vi "Dialog_TestBode (SubVI).vi"() -> ()   [LabVIEW 2017]
uses:
  <vilib>/Utility/miscctls.llb/LVRowAndColumnTypeDef.ctl
  Global_SNK3_HF.vi
panel:
  in  "Stop":bool
  in  "Clear":bool
  in  "FreqIndex":u32=46
  in  "FreqSel":bool
  in  "index":i32=11
  in  "Export":bool
  in  "Tab Control":enum32{"Page 1", "Page 2", "Page 3"}(tab)=enum."Page 2"
  in  "Table":string[][](table)=[["1.000000E+5", "1.000636E+5", "2.491840E-2"], ["1.120000E+5", "1.118741E+5", "3.785940E-2"], ["1.250000E+5", "1.249164E+5", "5.126945E-2"], ["1.400000E+5", "1.399830E+5", "6.506335E-2"], ["1.600000E+5", "1.599893E+5", "8.105153E-2"], ["1.800000E+5", "1.799900E+5", "9.492544E-2"], ["2.000000E+5", "1.999957E+5", "1.070040E-1"], ["2.240000E+5", "2.239947E+5", "1.194879E-1"], ["2.500000E+5", "2.499939E+5", "1.308049E-1"], ["2.800000E+5", "2.799909E+5", "1.415511E-1"], ["3.150000E+5", "3.149906E+5", "1.515264E-1"], ["3.550000E+5", "3.549888E+5", "1.604395E-1"], ["4.000000E+5", "3.999864E+5", "1.681297E-1"], ["4.500000E+5", "4.499863E+5", "1.745038E-1"], ["5.000000E+5", "4.999842E+5", "1.792983E-1"], ["5.600000E+5", "5.599829E+5", "1.838799E-1"], ["6.300000E+5", "6.299795E+5", "1.879248E-1"], ["7.100000E+5", "7.099802E+5", "1.908162E-1"], ["8.000000E+5", "7.999770E+5", "1.931713E-1"], ["9.000000E+5", "8.999726E+5", "1.950158E-1"], ["1.000000E+6", "9.999710E+5", "1.965268E-1"], ["1.120000E+6", "1.119965E+6", "1.976914E-1"], ["1.250000E+6", "1.249962E+6", "1.985237E-1"], ["1.400000E+6", "1.399956E+6", "1.991446E-1"], ["1.600000E+6", "1.599951E+6", "1.995656E-1"], ["1.800000E+6", "1.799943E+6", "1.997028E-1"], ["2.000000E+6", "1.999939E+6", "1.996953E-1"], ["2.240000E+6", "2.239928E+6", "1.994641E-1"], ["2.500000E+6", "2.499924E+6", "1.990983E-1"], ["2.800000E+6", "2.799912E+6", "1.985802E-1"], ["3.150000E+6", "3.149905E+6", "1.977598E-1"], ["3.550000E+6", "3.549890E+6", "1.967576E-1"], ["4.000000E+6", "3.999877E+6", "1.955042E-1"], ["4.500000E+6", "4.499864E+6", "1.940497E-1"], ["5.000000E+6", "4.999848E+6", "1.926097E-1"], ["5.600000E+6", "5.599830E+6", "1.907100E-1"], ["6.300000E+6", "6.299804E+6", "1.884695E-1"], ["7.100000E+6", "7.099783E+6", "1.857047E-1"], ["8.000000E+6", "7.999756E+6", "1.820427E-1"], ["9.000000E+6", "8.999724E+6", "1.769700E-1"], ["1.000000E+7", "9.999696E+6", "1.698254E-1"], ["1.120000E+7", "1.119966E+7", "1.575704E-1"], ["1.250000E+7", "1.249962E+7", "1.374566E-1"], ["1.400000E+7", "1.399957E+7", "1.010104E-1"], ["1.600000E+7", "1.599951E+7", "3.921273E-2"], ["1.800000E+7", "1.799945E+7", "7.166046E-3"], ["2.000000E+7", "1.999939E+7", "6.631099E-4"], ["1.000000E+5", "1.001610E+5", "2.507403E-2"], ["1.120000E+5", "1.118719E+5", "3.811099E-2"], ["1.250000E+5", "1.249126E+5", "5.159270E-2"], ["1.400000E+5", "1.399818E+5", "6.548660E-2"], ["1.600000E+5", "1.599863E+5", "8.150836E-2"], ["1.800000E+5", "1.799875E+5", "9.546910E-2"], ["2.000000E+5", "1.999953E+5", "1.076681E-1"], ["2.240000E+5", "2.239928E+5", "1.201877E-1"], ["2.500000E+5", "2.499918E+5", "1.316163E-1"], ["2.800000E+5", "2.799915E+5", "1.423784E-1"], ["3.150000E+5", "3.149935E+5", "1.525069E-1"], ["3.550000E+5", "3.549893E+5", "1.614557E-1"], ["4.000000E+5", "3.999897E+5", "1.690699E-1"], ["4.500000E+5", "4.499870E+5", "1.755943E-1"], ["5.000000E+5", "4.999845E+5", "1.803583E-1"], ["5.600000E+5", "5.599837E+5", "1.850528E-1"], ["6.300000E+5", "6.299822E+5", "1.891165E-1"], ["7.100000E+5", "7.099780E+5", "1.920091E-1"], ["8.000000E+5", "7.999766E+5", "1.943341E-1"], ["9.000000E+5", "8.999725E+5", "1.962455E-1"], ["1.000000E+6", "9.999694E+5", "1.977815E-1"], ["1.120000E+6", "1.119967E+6", "1.989120E-1"], ["1.250000E+6", "1.249961E+6", "1.997381E-1"], ["1.400000E+6", "1.399956E+6", "2.003866E-1"], ["1.600000E+6", "1.599951E+6", "2.008868E-1"], ["1.800000E+6", "1.799946E+6", "2.009867E-1"], ["2.000000E+6", "1.999937E+6", "2.010105E-1"], ["2.240000E+6", "2.239930E+6", "2.007797E-1"], ["2.500000E+6", "2.499926E+6", "2.004007E-1"], ["2.800000E+6", "2.799914E+6", "1.998448E-1"], ["3.150000E+6", "3.149906E+6", "1.990098E-1"], ["3.550000E+6", "3.549893E+6", "1.979898E-1"], ["4.000000E+6", "3.999878E+6", "1.966912E-1"], ["4.500000E+6", "4.499860E+6", "1.952348E-1"], ["5.000000E+6", "4.999849E+6", "1.936508E-1"], ["5.600000E+6", "5.599830E+6", "1.916568E-1"], ["6.300000E+6", "6.299805E+6", "1.893688E-1"], ["7.100000E+6", "7.099787E+6", "1.867505E-1"], ["8.000000E+6", "7.999758E+6", "1.838976E-1"], ["9.000000E+6", "8.999722E+6", "1.808635E-1"], ["1.000000E+7", "9.999696E+6", "1.777367E-1"], ["1.120000E+7", "1.119966E+7", "1.731531E-1"], ["1.250000E+7", "1.249962E+7", "1.649845E-1"], ["1.400000E+7", "1.399958E+7", "1.420928E-1"], ["1.600000E+7", "1.599951E+7", "7.711530E-2"], ["1.800000E+7", "1.799945E+7", "2.355849E-2"], ["2.000000E+7", "1.999939E+7", "4.626126E-3"], ["1.000000E+5", "1.001252E+5", "3.046975E-2"], ["1.120000E+5", "1.118759E+5", "4.637352E-2"], ["1.250000E+5", "1.249173E+5", "6.281049E-2"], ["1.400000E+5", "1.399846E+5", "7.988195E-2"], ["1.600000E+5", "1.599828E+5", "9.961572E-2"], ["1.800000E+5", "1.799853E+5", "1.168189E-1"], ["2.000000E+5", "1.999934E+5", "1.318127E-1"], ["2.240000E+5", "2.239952E+5", "1.473312E-1"], ["2.500000E+5", "2.499948E+5", "1.614577E-1"], ["2.800000E+5", "2.799918E+5", "1.749158E-1"], ["3.150000E+5", "3.149891E+5", "1.872912E-1"], ["3.550000E+5", "3.549888E+5", "1.983931E-1"], ["4.000000E+5", "3.999890E+5", "2.079678E-1"], ["4.500000E+5", "4.499874E+5", "2.159216E-1"], ["5.000000E+5", "4.999822E+5", "2.219795E-1"], ["5.600000E+5", "5.599815E+5", "2.277855E-1"], ["6.300000E+5", "6.299820E+5", "2.327026E-1"], ["7.100000E+5", "7.099788E+5", "2.362682E-1"], ["8.000000E+5", "7.999713E+5", "2.393311E-1"], ["9.000000E+5", "8.999711E+5", "2.416585E-1"], ["1.000000E+6", "9.999711E+5", "2.435690E-1"], ["1.120000E+6", "1.119965E+6", "2.450257E-1"], ["1.250000E+6", "1.249962E+6", "2.460204E-1"], ["1.400000E+6", "1.399956E+6", "2.467872E-1"], ["1.600000E+6", "1.599948E+6", "2.473571E-1"], ["1.800000E+6", "1.799945E+6", "2.475632E-1"], ["2.000000E+6", "1.999939E+6", "2.474866E-1"], ["2.240000E+6", "2.239933E+6", "2.470316E-1"], ["2.500000E+6", "2.499923E+6", "2.464084E-1"], ["2.800000E+6", "2.799913E+6", "2.454233E-1"], ["3.150000E+6", "3.149902E+6", "2.440672E-1"], ["3.550000E+6", "3.549894E+6", "2.421851E-1"], ["4.000000E+6", "3.999877E+6", "2.397798E-1"], ["4.500000E+6", "4.499864E+6", "2.368307E-1"], ["5.000000E+6", "4.999845E+6", "2.335615E-1"], ["5.600000E+6", "5.599827E+6", "2.292005E-1"], ["6.300000E+6", "6.299803E+6", "2.236615E-1"], ["7.100000E+6", "7.099783E+6", "2.165497E-1"], ["8.000000E+6", "7.999753E+6", "2.080278E-1"], ["9.000000E+6", "8.999724E+6", "1.978426E-1"], ["1.000000E+7", "9.999693E+6", "1.868804E-1"], ["1.120000E+7", "1.119965E+7", "1.725228E-1"], ["1.250000E+7", "1.249962E+7", "1.542881E-1"], ["1.400000E+7", "1.399957E+7", "1.237350E-1"], ["1.600000E+7", "1.599951E+7", "6.203397E-2"], ["1.800000E+7", "1.799944E+7", "1.812404E-2"], ["2.000000E+7", "1.999939E+7", "3.543936E-3"], ["1.000000E+5", "1.001588E+5", "2.947361E-2"], ["1.120000E+5", "1.118676E+5", "4.485788E-2"], ["1.250000E+5", "1.249118E+5", "6.086847E-2"], ["1.400000E+5", "1.399847E+5", "7.738364E-2"], ["1.600000E+5", "1.599909E+5", "9.659424E-2"], ["1.800000E+5", "1.799850E+5", "1.134125E-1"], ["2.000000E+5", "1.999928E+5", "1.281373E-1"], ["2.240000E+5", "2.239927E+5", "1.433162E-1"], ["2.500000E+5", "2.499955E+5", "1.571975E-1"], ["2.800000E+5", "2.799914E+5", "1.703684E-1"], ["3.150000E+5", "3.149886E+5", "1.827951E-1"], ["3.550000E+5", "3.549900E+5", "1.938016E-1"], ["4.000000E+5", "3.999887E+5", "2.034033E-1"], ["4.500000E+5", "4.499859E+5", "2.114272E-1"], ["5.000000E+5", "4.999831E+5", "2.175966E-1"], ["5.600000E+5", "5.599825E+5", "2.235053E-1"], ["6.300000E+5", "6.299793E+5", "2.287001E-1"], ["7.100000E+5", "7.099770E+5", "2.329029E-1"], ["8.000000E+5", "7.999752E+5", "2.365108E-1"], ["9.000000E+5", "8.999728E+5", "2.396521E-1"], ["1.000000E+6", "9.999702E+5", "2.422890E-1"], ["1.120000E+6", "1.119966E+6", "2.449885E-1"], ["1.250000E+6", "1.249961E+6", "2.474209E-1"], ["1.400000E+6", "1.399960E+6", "2.499920E-1"], ["1.600000E+6", "1.599951E+6", "2.531813E-1"], ["1.800000E+6", "1.799944E+6", "2.563808E-1"], ["2.000000E+6", "1.999939E+6", "2.597062E-1"], ["2.240000E+6", "2.239927E+6", "2.639021E-1"], ["2.500000E+6", "2.499924E+6", "2.688323E-1"], ["2.800000E+6", "2.799913E+6", "2.751680E-1"], ["3.150000E+6", "3.149904E+6", "2.834179E-1"], ["3.550000E+6", "3.549892E+6", "2.939424E-1"], ["4.000000E+6", "3.999879E+6", "3.073316E-1"], ["4.500000E+6", "4.499860E+6", "3.242399E-1"], ["5.000000E+6", "4.999846E+6", "3.430244E-1"], ["5.600000E+6", "5.599827E+6", "3.675444E-1"], ["6.300000E+6", "6.299807E+6", "3.977254E-1"], ["7.100000E+6", "7.099782E+6", "4.305227E-1"], ["8.000000E+6", "7.999753E+6", "4.582917E-1"], ["9.000000E+6", "8.999723E+6", "4.664814E-1"], ["1.000000E+7", "9.999692E+6", "4.421232E-1"], ["1.120000E+7", "1.119966E+7", "3.737524E-1"], ["1.250000E+7", "1.249961E+7", "2.750965E-1"], ["1.400000E+7", "1.399957E+7", "1.599110E-1"], ["1.600000E+7", "1.599950E+7", "4.612828E-2"], ["1.800000E+7", "1.799944E+7", "6.724351E-3"], ["2.000000E+7", "1.745191E+7", "5.547105E-4"], ["1.000000E+5", "1.001671E+5", "3.013311E-2"], ["1.120000E+5", "1.118716E+5", "4.587390E-2"], ["1.250000E+5", "1.249115E+5", "6.221882E-2"], ["1.400000E+5", "1.399901E+5", "7.910503E-2"], ["1.600000E+5", "1.599861E+5", "9.867014E-2"], ["1.800000E+5", "1.799875E+5", "1.157310E-1"], ["2.000000E+5", "1.999941E+5", "1.307408E-1"], ["2.240000E+5", "2.239941E+5", "1.461274E-1"], ["2.500000E+5", "2.499957E+5", "1.601914E-1"], ["2.800000E+5", "2.799922E+5", "1.735531E-1"], ["3.150000E+5", "3.149912E+5", "1.860088E-1"], ["3.550000E+5", "3.549891E+5", "1.971355E-1"], ["4.000000E+5", "3.999871E+5", "2.067383E-1"], ["4.500000E+5", "4.499858E+5", "2.147592E-1"], ["5.000000E+5", "4.999843E+5", "2.208970E-1"], ["5.600000E+5", "5.599830E+5", "2.267879E-1"], ["6.300000E+5", "6.299812E+5", "2.318491E-1"], ["7.100000E+5", "7.099781E+5", "2.356804E-1"], ["8.000000E+5", "7.999771E+5", "2.390532E-1"], ["9.000000E+5", "8.999704E+5", "2.418962E-1"], ["1.000000E+6", "9.999683E+5", "2.442224E-1"], ["1.120000E+6", "1.119965E+6", "2.463632E-1"], ["1.250000E+6", "1.249961E+6", "2.482126E-1"], ["1.400000E+6", "1.399956E+6", "2.498954E-1"], ["1.600000E+6", "1.599948E+6", "2.519791E-1"], ["1.800000E+6", "1.799946E+6", "2.538926E-1"], ["2.000000E+6", "1.999937E+6", "2.557256E-1"], ["2.240000E+6", "2.239932E+6", "2.579385E-1"], ["2.500000E+6", "2.499924E+6", "2.603118E-1"], ["2.800000E+6", "2.799913E+6", "2.634098E-1"], ["3.150000E+6", "3.149901E+6", "2.672305E-1"], ["3.550000E+6", "3.549891E+6", "2.720161E-1"], ["4.000000E+6", "3.999873E+6", "2.780268E-1"], ["4.500000E+6", "4.499860E+6", "2.852321E-1"], ["5.000000E+6", "4.999845E+6", "2.930384E-1"], ["5.600000E+6", "5.599826E+6", "3.028215E-1"], ["6.300000E+6", "6.299804E+6", "3.141354E-1"], ["7.100000E+6", "7.099781E+6", "3.257264E-1"], ["8.000000E+6", "7.999753E+6", "3.345783E-1"], ["9.000000E+6", "8.999721E+6", "3.357425E-1"], ["1.000000E+7", "9.999692E+6", "3.236355E-1"], ["1.120000E+7", "1.119965E+7", "2.898888E-1"], ["1.250000E+7", "1.249961E+7", "2.321748E-1"], ["1.400000E+7", "1.399957E+7", "1.483795E-1"], ["1.600000E+7", "1.599951E+7", "4.683820E-2"], ["1.800000E+7", "1.799944E+7", "7.169091E-3"], ["2.000000E+7", "1.999938E+7", "5.872768E-4"], ["1.000000E+5", "1.001573E+5", "3.042811E-2"], ["1.120000E+5", "1.118676E+5", "4.631044E-2"], ["1.250000E+5", "1.249112E+5", "6.278921E-2"], ["1.400000E+5", "1.399824E+5", "7.977333E-2"], ["1.600000E+5", "1.599897E+5", "9.949145E-2"], ["1.800000E+5", "1.799905E+5", "1.167352E-1"], ["2.000000E+5", "1.999960E+5", "1.317144E-1"], ["2.240000E+5", "2.239941E+5", "1.472570E-1"], ["2.500000E+5", "2.499914E+5", "1.614052E-1"], ["2.800000E+5", "2.799928E+5", "1.747607E-1"], ["3.150000E+5", "3.149895E+5", "1.872958E-1"], ["3.550000E+5", "3.549889E+5", "1.984372E-1"], ["4.000000E+5", "3.999899E+5", "2.080880E-1"], ["4.500000E+5", "4.499863E+5", "2.160420E-1"], ["5.000000E+5", "4.999824E+5", "2.221527E-1"], ["5.600000E+5", "5.599829E+5", "2.279609E-1"], ["6.300000E+5", "6.299811E+5", "2.329477E-1"], ["7.100000E+5", "7.099769E+5", "2.367245E-1"], ["8.000000E+5", "7.999745E+5", "2.398766E-1"], ["9.000000E+5", "8.999738E+5", "2.424630E-1"], ["1.000000E+6", "9.999694E+5", "2.445476E-1"], ["1.120000E+6", "1.119967E+6", "2.463587E-1"], ["1.250000E+6", "1.249961E+6", "2.477818E-1"], ["1.400000E+6", "1.399959E+6", "2.489776E-1"], ["1.600000E+6", "1.599947E+6", "2.503258E-1"], ["1.800000E+6", "1.799945E+6", "2.512193E-1"], ["2.000000E+6", "1.999942E+6", "2.520426E-1"], ["2.240000E+6", "2.239932E+6", "2.529437E-1"], ["2.500000E+6", "2.499923E+6", "2.538312E-1"], ["2.800000E+6", "2.799913E+6", "2.548656E-1"], ["3.150000E+6", "3.149903E+6", "2.559440E-1"], ["3.550000E+6", "3.549890E+6", "2.573163E-1"], ["4.000000E+6", "3.999877E+6", "2.589801E-1"], ["4.500000E+6", "4.499858E+6", "2.609782E-1"], ["5.000000E+6", "4.999846E+6", "2.630935E-1"], ["5.600000E+6", "5.599829E+6", "2.654121E-1"], ["6.300000E+6", "6.299805E+6", "2.678989E-1"], ["7.100000E+6", "7.099784E+6", "2.696164E-1"], ["8.000000E+6", "7.999755E+6", "2.688480E-1"], ["9.000000E+6", "8.999722E+6", "2.633041E-1"], ["1.000000E+7", "9.999690E+6", "2.505779E-1"], ["1.120000E+7", "1.119966E+7", "2.241202E-1"], ["1.250000E+7", "1.249961E+7", "1.824472E-1"], ["1.400000E+7", "1.399957E+7", "1.204614E-1"], ["1.600000E+7", "1.599951E+7", "4.016119E-2"], ["1.800000E+7", "1.799944E+7", "6.498026E-3"], ["2.000000E+7", "1.999938E+7", "5.582479E-4"], ["1.000000E+5", "1.001346E+5", "3.073302E-2"], ["1.120000E+5", "1.118727E+5", "4.677344E-2"], ["1.250000E+5", "1.249160E+5", "6.336208E-2"], ["1.400000E+5", "1.399837E+5", "8.046874E-2"], ["1.600000E+5", "1.599845E+5", "1.003864E-1"], ["1.800000E+5", "1.799893E+5", "1.177135E-1"], ["2.000000E+5", "1.999962E+5", "1.328408E-1"], ["2.240000E+5", "2.239946E+5", "1.484407E-1"], ["2.500000E+5", "2.499937E+5", "1.626519E-1"], ["2.800000E+5", "2.799899E+5", "1.761700E-1"], ["3.150000E+5", "3.149904E+5", "1.887583E-1"], ["3.550000E+5", "3.549888E+5", "1.998843E-1"], ["4.000000E+5", "3.999893E+5", "2.095560E-1"], ["4.500000E+5", "4.499866E+5", "2.176090E-1"], ["5.000000E+5", "4.999851E+5", "2.236199E-1"], ["5.600000E+5", "5.599840E+5", "2.295974E-1"], ["6.300000E+5", "6.299794E+5", "2.345735E-1"], ["7.100000E+5", "7.099800E+5", "2.382895E-1"], ["8.000000E+5", "7.999734E+5", "2.415122E-1"], ["9.000000E+5", "8.999709E+5", "2.440727E-1"], ["1.000000E+6", "9.999682E+5", "2.462285E-1"], ["1.120000E+6", "1.119965E+6", "2.480292E-1"], ["1.250000E+6", "1.249961E+6", "2.494651E-1"], ["1.400000E+6", "1.399958E+6", "2.506996E-1"], ["1.600000E+6", "1.599950E+6", "2.518965E-1"], ["1.800000E+6", "1.799947E+6", "2.529126E-1"], ["2.000000E+6", "1.999942E+6", "2.536920E-1"], ["2.240000E+6", "2.239931E+6", "2.547042E-1"], ["2.500000E+6", "2.499926E+6", "2.555771E-1"], ["2.800000E+6", "2.799914E+6", "2.565540E-1"], ["3.150000E+6", "3.149903E+6", "2.577524E-1"], ["3.550000E+6", "3.549891E+6", "2.590071E-1"], ["4.000000E+6", "3.999877E+6", "2.606799E-1"], ["4.500000E+6", "4.499863E+6", "2.625431E-1"], ["5.000000E+6", "4.999848E+6", "2.645213E-1"], ["5.600000E+6", "5.599827E+6", "2.667418E-1"], ["6.300000E+6", "6.299808E+6", "2.690356E-1"], ["7.100000E+6", "7.099784E+6", "2.709912E-1"], ["8.000000E+6", "7.999756E+6", "2.714708E-1"], ["9.000000E+6", "8.999725E+6", "2.690780E-1"], ["1.000000E+7", "9.999694E+6", "2.619751E-1"], ["1.120000E+7", "1.119966E+7", "2.461795E-1"], ["1.250000E+7", "1.249962E+7", "2.187268E-1"], ["1.400000E+7", "1.399957E+7", "1.694056E-1"], ["1.600000E+7", "1.599951E+7", "7.900056E-2"], ["1.800000E+7", "1.799946E+7", "2.134967E-2"], ["2.000000E+7", "1.999939E+7", "3.896080E-3"], ["1.000000E+5", "7.271622E+6", "3.725159E-4"], ["1.120000E+5", "8.112799E+6", "3.764415E-4"], ["1.250000E+5", "7.224727E+6", "3.662772E-4"], ["1.400000E+5", "7.308552E+6", "3.973020E-4"], ["1.600000E+5", "4.309535E+6", "3.626683E-4"], ["1.800000E+5", "6.453873E+6", "3.560410E-4"], ["2.000000E+5", "5.085443E+6", "3.513905E-4"], ["2.240000E+5", "7.989710E+6", "3.810558E-4"], ["2.500000E+5", "6.352418E+6", "3.677376E-4"], ["2.800000E+5", "7.506742E+6", "3.607153E-4"], ["3.150000E+5", "6.668509E+6", "3.890383E-4"], ["3.550000E+5", "6.895082E+6", "3.819765E-4"], ["4.000000E+5", "6.273636E+6", "3.413821E-4"], ["4.500000E+5", "6.840624E+6", "3.723358E-4"], ["5.000000E+5", "5.049030E+6", "3.681375E-4"], ["5.600000E+5", "6.333587E+6", "3.807082E-4"], ["6.300000E+5", "7.345420E+6", "3.871347E-4"], ["7.100000E+5", "7.099786E+5", "2.374579E-1"], ["8.000000E+5", "7.999729E+5", "2.406560E-1"], ["9.000000E+5", "8.999716E+5", "2.431850E-1"], ["1.000000E+6", "9.999691E+5", "2.451838E-1"], ["1.120000E+6", "1.119965E+6", "2.469041E-1"], ["1.250000E+6", "1.249961E+6", "2.482266E-1"], ["1.400000E+6", "1.399956E+6", "2.493007E-1"], ["1.600000E+6", "1.599949E+6", "2.503615E-1"], ["1.800000E+6", "1.799944E+6", "2.510987E-1"], ["2.000000E+6", "1.999940E+6", "2.517382E-1"], ["2.240000E+6", "2.239928E+6", "2.522363E-1"], ["2.500000E+6", "2.499921E+6", "2.527697E-1"], ["2.800000E+6", "2.799912E+6", "2.533518E-1"], ["3.150000E+6", "3.149900E+6", "2.538616E-1"], ["3.550000E+6", "3.549889E+6", "2.545760E-1"], ["4.000000E+6", "3.999879E+6", "2.551996E-1"], ["4.500000E+6", "4.499862E+6", "2.559211E-1"], ["5.000000E+6", "4.999847E+6", "2.566902E-1"], ["5.600000E+6", "5.599826E+6", "2.574986E-1"], ["6.300000E+6", "6.299806E+6", "2.578567E-1"], ["7.100000E+6", "7.099781E+6", "2.571842E-1"], ["8.000000E+6", "7.999755E+6", "2.542991E-1"], ["9.000000E+6", "8.999722E+6", "2.471375E-1"], ["1.000000E+7", "9.999692E+6", "2.341935E-1"], ["1.120000E+7", "1.119965E+7", "2.099252E-1"], ["1.250000E+7", "1.249961E+7", "1.724919E-1"], ["1.400000E+7", "1.399957E+7", "1.158079E-1"], ["1.600000E+7", "1.599951E+7", "3.952577E-2"], ["1.800000E+7", "1.799944E+7", "6.504605E-3"], ["2.000000E+7", "1.999938E+7", "5.650367E-4"], ["1.000000E+5", "1.001674E+5", "3.072473E-2"], ["1.120000E+5", "1.118718E+5", "4.674261E-2"], ["1.250000E+5", "1.249089E+5", "6.334272E-2"], ["1.400000E+5", "1.399846E+5", "8.047815E-2"], ["1.600000E+5", "1.599821E+5", "1.003712E-1"], ["1.800000E+5", "1.799898E+5", "1.176893E-1"], ["2.000000E+5", "1.999934E+5", "1.327762E-1"], ["2.240000E+5", "2.239896E+5", "1.483583E-1"], ["2.500000E+5", "2.499930E+5", "1.626360E-1"], ["2.800000E+5", "2.799919E+5", "1.760684E-1"], ["3.150000E+5", "3.149892E+5", "1.886214E-1"], ["3.550000E+5", "3.549895E+5", "1.997476E-1"], ["4.000000E+5", "3.999900E+5", "2.094032E-1"], ["4.500000E+5", "4.499880E+5", "2.174488E-1"], ["5.000000E+5", "4.999829E+5", "2.235411E-1"], ["5.600000E+5", "5.599852E+5", "2.293669E-1"], ["6.300000E+5", "6.299816E+5", "2.344044E-1"], ["7.100000E+5", "7.099792E+5", "2.380854E-1"], ["8.000000E+5", "7.999787E+5", "2.411883E-1"], ["9.000000E+5", "8.999727E+5", "2.436654E-1"], ["1.000000E+6", "9.999702E+5", "2.457231E-1"], ["1.120000E+6", "1.119968E+6", "2.474353E-1"], ["1.250000E+6", "1.249962E+6", "2.487468E-1"], ["1.400000E+6", "1.399959E+6", "2.498615E-1"], ["1.600000E+6", "1.599952E+6", "2.508693E-1"], ["1.800000E+6", "1.799943E+6", "2.517389E-1"], ["2.000000E+6", "1.999941E+6", "2.522760E-1"], ["2.240000E+6", "2.239933E+6", "2.527969E-1"], ["2.500000E+6", "2.499923E+6", "2.533575E-1"], ["2.800000E+6", "2.799916E+6", "2.538892E-1"], ["3.150000E+6", "3.149903E+6", "2.544033E-1"], ["3.550000E+6", "3.549890E+6", "2.550274E-1"], ["4.000000E+6", "3.999878E+6", "2.557525E-1"], ["4.500000E+6", "4.499865E+6", "2.565297E-1"], ["5.000000E+6", "4.999845E+6", "2.572363E-1"], ["5.600000E+6", "5.599828E+6", "2.580387E-1"], ["6.300000E+6", "6.299804E+6", "2.584150E-1"], ["7.100000E+6", "7.099784E+6", "2.577035E-1"], ["8.000000E+6", "7.999757E+6", "2.547739E-1"], ["9.000000E+6", "8.999726E+6", "2.475172E-1"], ["1.000000E+7", "9.999692E+6", "2.346899E-1"], ["1.120000E+7", "1.119966E+7", "2.102803E-1"], ["1.250000E+7", "1.249962E+7", "1.727500E-1"], ["1.400000E+7", "1.399957E+7", "1.159860E-1"], ["1.600000E+7", "1.599951E+7", "3.956788E-2"], ["1.800000E+7", "1.799945E+7", "6.511833E-3"], ["2.000000E+7", "1.999939E+7", "5.656747E-4"], ["1.000000E+5", "4.945255E+6", "3.784724E-4"], ["1.120000E+5", "6.375661E+6", "3.745710E-4"], ["1.250000E+5", "1.250073E+5", "6.132748E-4"], ["1.400000E+5", "1.399781E+5", "1.172522E-3"], ["1.600000E+5", "1.600019E+5", "2.449967E-3"], ["1.800000E+5", "1.799905E+5", "4.581770E-3"], ["2.000000E+5", "1.999999E+5", "7.885116E-3"], ["2.240000E+5", "2.240013E+5", "1.387170E-2"], ["2.500000E+5", "2.499991E+5", "2.357577E-2"], ["2.800000E+5", "2.799918E+5", "3.982715E-2"], ["3.150000E+5", "3.149929E+5", "6.635508E-2"], ["3.550000E+5", "3.549946E+5", "1.045620E-1"], ["4.000000E+5", "3.999874E+5", "1.487510E-1"], ["4.500000E+5", "4.499825E+5", "1.863709E-1"], ["5.000000E+5", "4.999817E+5", "2.090956E-1"], ["5.600000E+5", "5.599827E+5", "2.239868E-1"], ["6.300000E+5", "6.299815E+5", "2.330744E-1"], ["7.100000E+5", "7.099780E+5", "2.383611E-1"], ["8.000000E+5", "7.999752E+5", "2.420167E-1"], ["9.000000E+5", "8.999734E+5", "2.447763E-1"], ["1.000000E+6", "9.999693E+5", "2.468706E-1"], ["1.120000E+6", "1.119966E+6", "2.485843E-1"], ["1.250000E+6", "1.249960E+6", "2.498993E-1"], ["1.400000E+6", "1.399960E+6", "2.509156E-1"], ["1.600000E+6", "1.599954E+6", "2.521203E-1"], ["1.800000E+6", "1.799947E+6", "2.528407E-1"], ["2.000000E+6", "1.999941E+6", "2.534274E-1"], ["2.240000E+6", "2.239932E+6", "2.540286E-1"], ["2.500000E+6", "2.499922E+6", "2.545439E-1"], ["2.800000E+6", "2.799913E+6", "2.550617E-1"], ["3.150000E+6", "3.149905E+6", "2.555762E-1"], ["3.550000E+6", "3.549890E+6", "2.562070E-1"], ["4.000000E+6", "3.999879E+6", "2.568503E-1"], ["4.500000E+6", "4.499863E+6", "2.576394E-1"], ["5.000000E+6", "4.999848E+6", "2.583673E-1"], ["5.600000E+6", "5.599828E+6", "2.590441E-1"], ["6.300000E+6", "6.299811E+6", "2.594208E-1"], ["7.100000E+6", "7.099782E+6", "2.587419E-1"], ["8.000000E+6", "7.999757E+6", "2.556978E-1"], ["9.000000E+6", "8.999729E+6", "2.484300E-1"], ["1.000000E+7", "9.999696E+6", "2.355078E-1"], ["1.120000E+7", "1.119966E+7", "2.112248E-1"], ["1.250000E+7", "1.249962E+7", "1.739360E-1"], ["1.400000E+7", "1.399957E+7", "1.167797E-1"], ["1.600000E+7", "1.599951E+7", "3.926693E-2"], ["1.800000E+7", "1.799945E+7", "6.325551E-3"], ["2.000000E+7", "1.999939E+7", "5.422671E-4"], ["1.000000E+5", "6.172924E+6", "3.758029E-4"], ["1.120000E+5", "5.205844E+6", "3.767627E-4"], ["1.250000E+5", "1.250007E+5", "6.162397E-4"], ["1.400000E+5", "1.399804E+5", "1.177858E-3"], ["1.600000E+5", "1.600003E+5", "2.461317E-3"], ["1.800000E+5", "1.799938E+5", "4.602202E-3"], ["2.000000E+5", "2.000005E+5", "7.917076E-3"], ["2.240000E+5", "2.239992E+5", "1.394228E-2"], ["2.500000E+5", "2.499997E+5", "2.367325E-2"], ["2.800000E+5", "2.799971E+5", "4.000153E-2"], ["3.150000E+5", "3.149938E+5", "6.665400E-2"], ["3.550000E+5", "3.549936E+5", "1.050529E-1"], ["4.000000E+5", "3.999878E+5", "1.493885E-1"], ["4.500000E+5", "4.499854E+5", "1.871373E-1"], ["5.000000E+5", "4.999850E+5", "2.099204E-1"], ["5.600000E+5", "5.599840E+5", "2.249705E-1"], ["6.300000E+5", "6.299796E+5", "2.340463E-1"], ["7.100000E+5", "7.099780E+5", "2.393587E-1"], ["8.000000E+5", "7.999747E+5", "2.431090E-1"], ["9.000000E+5", "8.999714E+5", "2.458491E-1"], ["1.000000E+6", "9.999705E+5", "2.479870E-1"], ["1.120000E+6", "1.119964E+6", "2.496587E-1"], ["1.250000E+6", "1.249962E+6", "2.510589E-1"], ["1.400000E+6", "1.399958E+6", "2.521599E-1"], ["1.600000E+6", "1.599952E+6", "2.532737E-1"], ["1.800000E+6", "1.799945E+6", "2.541091E-1"], ["2.000000E+6", "1.999939E+6", "2.546832E-1"], ["2.240000E+6", "2.239931E+6", "2.552231E-1"], ["2.500000E+6", "2.499922E+6", "2.557674E-1"], ["2.800000E+6", "2.799916E+6", "2.562845E-1"], ["3.150000E+6", "3.149902E+6", "2.569137E-1"], ["3.550000E+6", "3.549892E+6", "2.574992E-1"], ["4.000000E+6", "3.999881E+6", "2.581088E-1"], ["4.500000E+6", "4.499866E+6", "2.587312E-1"], ["5.000000E+6", "4.999849E+6", "2.594061E-1"], ["5.600000E+6", "5.599830E+6", "2.599108E-1"], ["6.300000E+6", "6.299809E+6", "2.602532E-1"], ["7.100000E+6", "7.099784E+6", "2.598564E-1"], ["8.000000E+6", "7.999759E+6", "2.578969E-1"], ["9.000000E+6", "8.999725E+6", "2.536606E-1"], ["1.000000E+7", "9.999695E+6", "2.460182E-1"], ["1.120000E+7", "1.119966E+7", "2.318706E-1"], ["1.250000E+7", "1.249962E+7", "2.082904E-1"], ["1.400000E+7", "1.399957E+7", "1.640904E-1"], ["1.600000E+7", "1.599951E+7", "7.713568E-2"], ["1.800000E+7", "1.799945E+7", "2.076200E-2"], ["2.000000E+7", "1.999939E+7", "3.781710E-3"]]
  out "XY Graph - Light":cluster{dbl[], dbl[]}[](graph)=[{[100000.0], [-32.06959712907717]}, {[111999.99999999999, 125000.0, 140000.0, 160000.0, 180000.0, 200000.0, 223999.99999999997, 250000.0, 280000.0, 315000.0, 355000.0, 400000.0, 450000.0, 500000.0, 560000.0, 630000.0, 710000.0, 800000.0, 900000.0, 1000000.0, 1119999.9999999998, 1250000.0, 1400000.0, 1600000.0, 1800000.0, 2000000.0, 2239999.9999999995, 2500000.0, 2800000.0, 3150000.0, 3550000.0, 4000000.0, 4500000.0, 5000000.0, 5600000.0, 6300000.0, 7100000.0, 8000000.0, 9000000.0, 10000000.0, 11199999.999999998, 12500000.0, 14000000.0, 16000000.0, 18000000.0, 20000000.0], [-28.436526298205948, -25.802826263296893, -23.7332719575054, -21.82477578258775, -20.452347258891514, -19.412002724486356, -18.45351884411941, -17.667519012682238, -16.98173568676242, -16.390231995354895, -15.893775113201198, -15.487111701662231, -15.16390087209189, -14.928475216865047, -14.709313208203444, -14.52032036334469, -14.387693344743568, -14.281150043223814, -14.198605408554283, -14.131565591838937, -14.08024587698728, -14.043750917215725, -14.016628526957223, -13.998285225401968, -13.992317823456125, -13.992641918238395, -14.002703149579682, -14.018650076231129, -14.04128269413424, -14.077239595490907, -14.121370204146462, -14.176878604262049, -14.241741662590712, -14.306437043319807, -14.392531267070934, -14.495179556946546, -14.623544203236058, -14.796536706787954, -15.042006383001034, -15.399947629850084, -16.050507306854122, -17.23668939060284, -19.912677810583506, -28.131459030407164, -42.89440763935011, -63.56829035942]}, {[100000.0, 111999.99999999999, 125000.0, 140000.0, 160000.0, 180000.0, 200000.0, 223999.99999999997, 250000.0, 280000.0, 315000.0, 355000.0, 400000.0, 450000.0, 500000.0, 560000.0, 630000.0, 710000.0, 800000.0, 900000.0, 1000000.0, 1119999.9999999998, 1250000.0, 1400000.0, 1600000.0, 1800000.0, 2000000.0, 2239999.9999999995, 2500000.0, 2800000.0, 3150000.0, 3550000.0, 4000000.0, 4500000.0, 5000000.0, 5600000.0, 6300000.0, 7100000.0, 8000000.0, 9000000.0, 10000000.0, 11199999.999999998, 12500000.0, 14000000.0, 16000000.0, 18000000.0, 20000000.0], [-32.01551889429962, -28.37899452707971, -25.74823483212413, -23.676951031879764, -21.77595640844784, -20.40274326154021, -19.358259454411325, -18.402801613986824, -17.613805446903246, -16.93111990056153, -16.33421225385209, -15.838929891678752, -15.438674054644316, -15.109793842110058, -14.877276187309834, -14.65408910002438, -14.46541001449438, -14.333564100378442, -14.2290213916183, -14.144008009132534, -14.076285861022662, -14.026778773392161, -13.990782390455067, -13.962626095388547, -13.940972167945166, -13.936653414445281, -13.93562605041957, -13.945605110001921, -13.962017482691687, -13.986141635395718, -14.022512471882182, -14.067143854670874, -14.124299218352473, -14.188853652759148, -14.259612495960825, -14.349517323308962, -14.453830406996547, -14.574765674860101, -14.708480691090395, -14.852983060476303, -15.004455418435583, -15.23139293918094, -15.651137537678274, -16.948557340120082, -22.257188494263005, -32.557051745684504, -46.69565079423197]}, {[100000.0, 111999.99999999999, 125000.0, 140000.0, 160000.0, 180000.0, 200000.0, 223999.99999999997, 250000.0, 280000.0, 315000.0, 355000.0, 400000.0, 450000.0, 500000.0, 560000.0, 630000.0, 710000.0, 800000.0, 900000.0, 1000000.0, 1119999.9999999998, 1250000.0, 1400000.0, 1600000.0, 1800000.0, 2000000.0, 2239999.9999999995, 2500000.0, 2800000.0, 3150000.0, 3550000.0, 4000000.0, 4500000.0, 5000000.0, 5600000.0, 6300000.0, 7100000.0, 8000000.0, 9000000.0, 10000000.0, 11199999.999999998, 12500000.0, 14000000.0, 16000000.0, 18000000.0, 20000000.0], [-30.322621218434477, -26.674599312380135, -24.039355742967786, -21.951026345450444, -20.033442386519425, -18.64973877846673, -17.600856535055836, -16.63410559857063, -15.83882726130537, -15.143417277389128, -14.549652554538168, -14.049467339340184, -13.6400770187213, -13.314077380890701, -13.073743856192044, -12.849477273241554, -12.663977095040204, -12.531894145111133, -12.420015799221297, -12.33595721749724, -12.267560469194702, -12.215768532393055, -12.180579015082117, -12.153546074218175, -12.133510861761497, -12.12627824947159, -12.128967694603269, -12.144950624208512, -12.166889105606614, -12.201685155510308, -12.249811738460137, -12.317053271217207, -12.403748427428795, -12.511239170989356, -12.631974094798718, -12.795689318081582, -13.008175123698402, -13.288846918372247, -13.637571959268593, -14.073604548608769, -14.56872406173578, -15.26306825122991, -16.233350560286397, -18.150148684410517, -24.147407966054967, -34.83489953792064, -49.010283136140494]}, {[100000.0, 111999.99999999999, 125000.0, 140000.0, 160000.0, 180000.0, 200000.0, 223999.99999999997, 250000.0, 280000.0, 315000.0, 355000.0, 400000.0, 450000.0, 500000.0, 560000.0, 630000.0, 710000.0, 800000.0, 900000.0, 1000000.0, 1119999.9999999998, 1250000.0, 1400000.0, 1600000.0, 1800000.0, 2000000.0, 2239999.9999999995, 2500000.0, 2800000.0, 3150000.0, 3550000.0, 4000000.0, 4500000.0, 5000000.0, 5600000.0, 6300000.0, 7100000.0, 8000000.0, 9000000.0, 10000000.0, 11199999.999999998, 12500000.0, 14000000.0, 16000000.0, 18000000.0, 20000000.0], [-30.61133369738789, -26.963226015672408, -24.312152300260493, -22.22701720360909, -20.30097563747857, -18.90678532691976, -17.846487376256462, -16.874093584233275, -16.071085496798904, -15.372220087819837, -14.760709193608438, -14.252851833614361, -13.832841107089678, -13.496784135647319, -13.246958490658088, -13.01424181279698, -12.81467178595403, -12.656501341972826, -12.522979917934427, -12.408375492365128, -12.313327623976056, -12.21708601380307, -12.131271682782272, -12.04147663588503, -11.931368786082132, -11.822288890386137, -11.710354665088174, -11.571143527779846, -11.410370324688335, -11.208041474378902, -10.951453674000465, -10.634756112896229, -10.247856230096259, -9.782671188369868, -9.293500006339334, -8.69380341275508, -8.008333928935542, -7.320078807085363, -6.777160551500607, -6.623312531960201, -7.089134809418943, -8.548319619608288, -11.21029715297354, -15.922431897186373, -26.720654327600442, -43.446992917597, -65.11867214507339]}, {[100000.0, 111999.99999999999, 125000.0, 140000.0, 160000.0, 180000.0, 200000.0, 223999.99999999997, 250000.0, 280000.0, 315000.0, 355000.0, 400000.0, 450000.0, 500000.0, 560000.0, 630000.0, 710000.0, 800000.0, 900000.0, 1000000.0, 1119999.9999999998, 1250000.0, 1400000.0, 1600000.0, 1800000.0, 2000000.0, 2239999.9999999995, 2500000.0, 2800000.0, 3150000.0, 3550000.0, 4000000.0, 4500000.0, 5000000.0, 5600000.0, 6300000.0, 7100000.0, 8000000.0, 9000000.0, 10000000.0, 11199999.999999998, 12500000.0, 14000000.0, 16000000.0, 18000000.0, 20000000.0], [-30.41912035321658, -26.768686854286035, -24.121564852930433, -22.035918034919998, -20.11628492359509, -18.731007508690304, -17.67178020513984, -16.705366019589768, -15.907216887832798, -15.21135159574845, -14.609327938842513, -14.10470130853527, -13.691582339358213, -13.360964284671827, -13.116205469885676, -12.887600720975048, -12.695892003681614, -12.553529436783348, -12.430110309952902, -12.32741743046304, -12.244288567857806, -12.168483384389607, -12.103522164856294, -12.044833880465378, -11.972709681316775, -11.907000406404599, -11.844515582541694, -11.769675619461665, -11.690123894865298, -11.587361772358634, -11.462278975379236, -11.308107441500576, -11.118265772506817, -10.896031225741762, -10.661508462404504, -10.376264686527499, -10.057661589904734, -9.742940895315584, -9.510045715933911, -9.479873007304905, -9.798877177842863, -10.755370700425487, -12.683696600970704, -16.57252108145334, -26.587996933968444, -42.8907183233943, -64.62314271153984]}, {[100000.0, 111999.99999999999, 125000.0, 140000.0, 160000.0, 180000.0, 200000.0, 223999.99999999997, 250000.0, 280000.0, 315000.0, 355000.0, 400000.0, 450000.0, 500000.0, 560000.0, 630000.0, 710000.0, 800000.0, 900000.0, 1000000.0, 1119999.9999999998, 1250000.0, 1400000.0, 1600000.0, 1800000.0, 2000000.0, 2239999.9999999995, 2500000.0, 2800000.0, 3150000.0, 3550000.0, 4000000.0, 4500000.0, 5000000.0, 5600000.0, 6300000.0, 7100000.0, 8000000.0, 9000000.0, 10000000.0, 11199999.999999998, 12500000.0, 14000000.0, 16000000.0, 18000000.0, 20000000.0], [-30.33450156596599, -26.686421458352868, -24.042299781442434, -21.96284517278093, -20.04428464259955, -18.655966429280745, -17.60733470043496, -16.638479338035044, -15.841648411980444, -15.15112442170788, -14.549438867976725, -14.047538572712, -13.635058488279245, -13.309234710302002, -13.066969241980635, -12.84279115991943, -12.654833198920299, -12.515134570073972, -12.400243590644633, -12.30709032840063, -12.232731212616173, -12.168643308975236, -12.118612808408507, -12.07679605908064, -12.02988614388056, -11.998938644551348, -11.970521047293492, -11.939523834626698, -11.909099785768307, -11.873774674735621, -11.83710084124488, -11.790653095959714, -11.734672393853796, -11.667914202761203, -11.597796461965483, -11.521584980850847, -11.440581004281576, -11.38507545220435, -11.409864067646199, -11.590848492118708, -12.021146340221676, -12.990378844603033, -14.777256627783688, -18.383044645435472, -27.923869003228216, -43.744371659949636, -65.06345806592672]}, {[100000.0, 111999.99999999999, 125000.0, 140000.0, 160000.0, 180000.0, 200000.0, 223999.99999999997, 250000.0, 280000.0, 315000.0, 355000.0, 400000.0, 450000.0, 500000.0, 560000.0, 630000.0, 710000.0, 800000.0, 900000.0, 1000000.0, 1119999.9999999998, 1250000.0, 1400000.0, 1600000.0, 1800000.0, 2000000.0, 2239999.9999999995, 2500000.0, 2800000.0, 3150000.0, 3550000.0, 4000000.0, 4500000.0, 5000000.0, 5600000.0, 6300000.0, 7100000.0, 8000000.0, 9000000.0, 10000000.0, 11199999.999999998, 12500000.0, 14000000.0, 16000000.0, 18000000.0, 20000000.0], [-30.24789404996484, -26.600013883835068, -23.96341201143198, -21.887456100748853, -19.966499876121567, -18.583473412311562, -17.53337202480331, -16.56893935297809, -15.774819618881704, -15.081361718428841, -14.481877791316837, -13.984427538167008, -13.573997983159764, -13.246461065447326, -13.009789862233173, -12.780660526050575, -12.594421135111038, -12.457902957012859, -12.341218848368996, -12.24961431316909, -12.173232020991197, -12.109943123673748, -12.059802499359078, -12.016926245042542, -11.975558229560114, -11.940591311807667, -11.913862881998543, -11.879277879830017, -11.849560012160229, -11.816423207019596, -11.775944007511054, -11.733765384826949, -11.67785014492784, -11.615987282648316, -11.550785921942488, -11.47817897419219, -11.403803588623836, -11.340896181601586, -11.325538191069693, -11.402436420707907, -11.63479852536646, -12.174961172364398, -13.201960511258275, -15.421446391245556, -22.047396531216165, -33.4121769345505, -48.18744198752221]}, {[100000.0, 111999.99999999999, 125000.0, 140000.0, 160000.0, 180000.0, 200000.0, 223999.99999999997, 250000.0, 280000.0, 315000.0, 355000.0, 400000.0, 450000.0, 500000.0, 560000.0, 630000.0, 710000.0, 800000.0, 900000.0, 1000000.0, 1119999.9999999998, 1250000.0, 1400000.0, 1600000.0, 1800000.0, 2000000.0, 2239999.9999999995, 2500000.0, 2800000.0, 3150000.0, 3550000.0, 4000000.0, 4500000.0, 5000000.0, 5600000.0, 6300000.0, 7100000.0, 8000000.0, 9000000.0, 10000000.0, 11199999.999999998, 12500000.0, 14000000.0, 16000000.0, 18000000.0, 20000000.0], [-68.57710357690299, -68.48605116826893, -68.72380263693235, -68.01758533621042, -68.80980892885557, -68.96999899981928, -69.08420034725333, -68.38022834982722, -68.68924011743366, -68.85670925472124, -68.2001525136999, -68.3592667376062, -69.33518529957286, -68.58130425925606, -68.67979817145846, -68.38815634294961, -68.24275797773083, -12.488266184754659, -12.372065992373845, -12.281263018915336, -12.210163933420446, -12.149434619017462, -12.103034536863998, -12.065528732359056, -12.028648304823495, -12.003110944042156, -11.981019272008659, -11.963848285615535, -11.945498696424583, -11.92551885961441, -11.908059089189912, -11.88365060133041, -11.862401062413017, -11.837876814313525, -11.811813414511331, -11.784501952989414, -11.772432981013141, -11.795113130633561, -11.893103376612657, -12.141225988677553, -12.608502827899795, -13.558708826225732, -15.264628063371308, -18.7252370168565, -28.062393488061264, -43.735581168552315, -64.95846637089771]}, {[100000.0, 111999.99999999999, 125000.0, 140000.0, 160000.0, 180000.0, 200000.0, 223999.99999999997, 250000.0, 280000.0, 315000.0, 355000.0, 400000.0, 450000.0, 500000.0, 560000.0, 630000.0, 710000.0, 800000.0, 900000.0, 1000000.0, 1119999.9999999998, 1250000.0, 1400000.0, 1600000.0, 1800000.0, 2000000.0, 2239999.9999999995, 2500000.0, 2800000.0, 3150000.0, 3550000.0, 4000000.0, 4500000.0, 5000000.0, 5600000.0, 6300000.0, 7100000.0, 8000000.0, 9000000.0, 10000000.0, 11199999.999999998, 12500000.0, 14000000.0, 16000000.0, 18000000.0, 20000000.0], [-30.250238600547323, -26.60574123305218, -23.966065826769682, -21.88644004674048, -19.967815248866582, -18.585258261555133, -17.537596663834936, -16.57376587443311, -15.775666913529545, -15.086369873908755, -14.488179619572058, -13.99036930964199, -13.58033536381768, -13.252859433681968, -13.012850812133351, -12.789385956800812, -12.600684971598024, -12.465345817110727, -12.352874240424248, -12.2641215351186, -12.191080105325087, -12.130767559284411, -12.084848657947054, -12.046012147360676, -12.011048947677141, -11.980991811439626, -11.962479660520648, -11.944564946667013, -11.925323065929481, -11.90711491020946, -11.889544986186607, -11.868263037254064, -11.843603692408573, -11.817245800439345, -11.793356255749707, -11.766303562318965, -11.753647227477156, -11.777595147044327, -11.876900973792461, -12.12789361931333, -12.590110517643126, -13.544029834199758, -15.25163902565762, -18.711890411343116, -28.053143292588395, -43.725935554124376, -64.94866486618284]}, {[100000.0, 111999.99999999999, 125000.0, 140000.0, 160000.0, 180000.0, 200000.0, 223999.99999999997, 250000.0, 280000.0, 315000.0, 355000.0, 400000.0, 450000.0, 500000.0, 560000.0, 630000.0, 710000.0, 800000.0, 900000.0, 1000000.0, 1119999.9999999998, 1250000.0, 1400000.0, 1600000.0, 1800000.0, 2000000.0, 2239999.9999999995, 2500000.0, 2800000.0, 3150000.0, 3550000.0, 4000000.0, 4500000.0, 5000000.0, 5600000.0, 6300000.0, 7100000.0, 8000000.0, 9000000.0, 10000000.0, 11199999.999999998, 12500000.0, 14000000.0, 16000000.0, 18000000.0, 20000000.0], [-68.43931520457295, -68.52931584348254, -64.2468969064375, -58.61757829042208, -52.21679666976928, -46.77933503497029, -42.06383776297401, -37.157408809543796, -32.550683409950835, -27.996414600540803, -23.562516698228112, -19.61252287178319, -16.55080381291166, -14.592436013839977, -13.593103990901279, -12.995551237745502, -12.650109604937398, -12.455293699033605, -12.323093326225653, -12.22461317189081, -12.150610805258768, -12.090526308319308, -12.044699167449362, -12.00944642925072, -11.967845261220166, -11.9430612233058, -11.922928048913965, -11.902347948459473, -11.884745222195026, -11.867094030053675, -11.84959209979203, -11.828180850388737, -11.806397008114075, -11.779753111439248, -11.75524800263961, -11.73252556651821, -11.719903930861657, -11.74266507839108, -11.845460366356047, -12.095917730516359, -12.559892999319795, -13.505102231447202, -15.192209489908109, -18.652656522969846, -28.11946188915508, -43.978033207370615, -65.31573537349254]}, {[100000.0, 111999.99999999999, 125000.0, 140000.0, 160000.0, 180000.0, 200000.0, 223999.99999999997, 250000.0, 280000.0, 315000.0, 355000.0, 400000.0, 450000.0, 500000.0, 560000.0, 630000.0, 710000.0, 800000.0, 900000.0, 1000000.0, 1119999.9999999998, 1250000.0, 1400000.0, 1600000.0, 1800000.0, 2000000.0, 2239999.9999999995, 2500000.0, 2800000.0, 3150000.0, 3550000.0, 4000000.0, 4500000.0, 5000000.0, 5600000.0, 6300000.0, 7100000.0, 8000000.0, 9000000.0, 10000000.0, 11199999.999999998, 12500000.0, 14000000.0, 16000000.0, 18000000.0, 20000000.0], [-68.50079763226556, -68.47864197543183, -64.20500696831749, -58.57813928928698, -52.1766496150407, -46.74068717461809, -42.028703394267026, -37.113326999091846, -32.514842899141904, -27.95846823508784, -23.523475743601562, -19.571837940730948, -16.51365429054962, -14.556794185838964, -13.558906052814852, -12.957487506163293, -12.61396429182807, -12.41901495709101, -12.283978084001191, -12.186626529098115, -12.111423183431821, -12.053065578005446, -12.00448719202477, -11.966477944223342, -11.92819889683417, -11.899596516182152, -11.879994926881869, -11.861600155863155, -11.84309693794751, -11.825553378217624, -11.804254944805441, -11.78448213944315, -11.763945210842051, -11.743024246527858, -11.72039542479753, -11.703512317421653, -11.692077361374768, -11.705330299747258, -11.771076923700072, -11.914940479423539, -12.180655159814966, -12.695084974193563, -13.62661537871501, -15.69833431052672, -22.25489328671155, -33.65461483440774, -48.44623497916292]}]
  in  "Генератор":refnum<visa-resource-name>="USB0::0x164E::0x0FA1::TW00009918::INSTR"
  out "FFT amplitude":dbl=0.0037817102532093612
  out "detected frequency":dbl=19999391.662828922
  out "FreqArray":dbl[](array[numeric])=[100000.0, 111999.99999999999, 125000.0, 140000.0, 160000.0, 180000.0, 200000.0, 223999.99999999997, 250000.0, 280000.0, 315000.0, 355000.0, 400000.0, 450000.0, 500000.0, 560000.0, 630000.0, 710000.0, 800000.0, 900000.0, 1000000.0, 1119999.9999999998, 1250000.0, 1400000.0, 1600000.0, 1800000.0, 2000000.0, 2239999.9999999995, 2500000.0, 2800000.0, 3150000.0, 3550000.0, 4000000.0, 4500000.0, 5000000.0, 5600000.0, 6300000.0, 7100000.0, 8000000.0, 9000000.0, 10000000.0, 11199999.999999998, 12500000.0, 14000000.0, 16000000.0, 18000000.0, 20000000.0]
  out "FREQuency":string="20000000.000000"
  in  "VOLTage":string="0.317"
  out "ConnectedGen":bool caption="Генерато подключен"
  out "readGen":string="PRIST CORP.,AKIP-3402,TW00009918,2.09-0B2-04-03-04\n"
  in  "GenCon":bool
  out "FreqCurrent":dbl=20000000.0 format="%#_6p"
  in  "Stop":bool
  in  "Ring":u16(ring) items=["ПЭП1...ПЭП8", "ПЭП9...ПЭП16"]
  out "MeasProcces":bool
  out "MeasStart":u32=24277382
  in  "MeasPause":u32=1000
  in  "StartMeas":bool
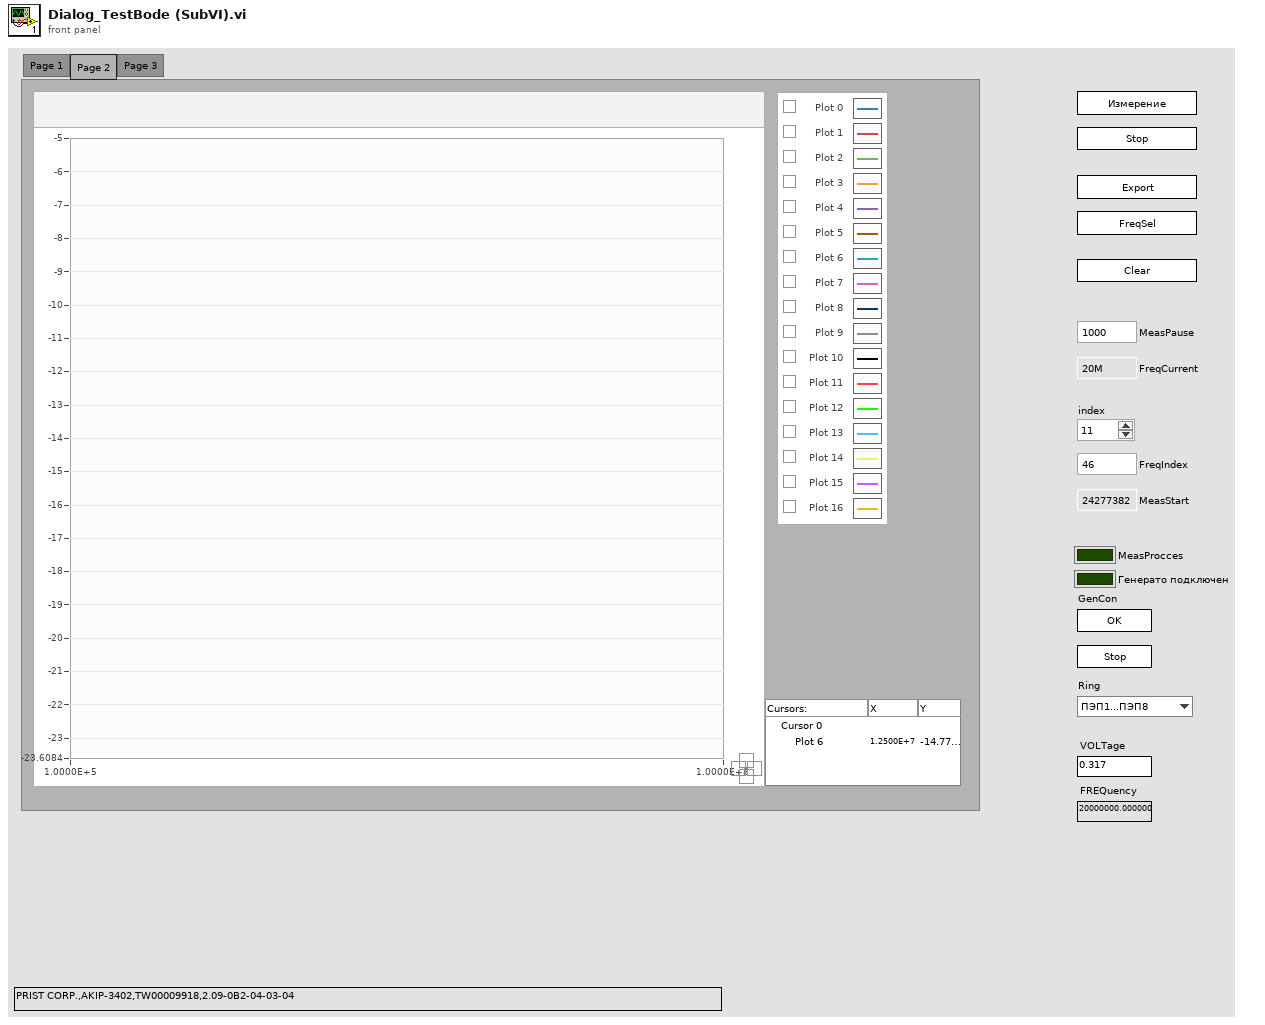
[diagram p1: front panel]
types:
  T1 = typedef "LVRowAndColumnTypeDef.ctl" = cluster{"Row":i32, "Column":i32}
  T2 = typedef "MeasControl.ctl" = cluster{"FFT amplitude":dbl, "amplitude":dbl, "RMS":dbl, "detected frequency":dbl, "way sensor 1":ext, "way sensor 2":ext, "detected frequency 2":dbl, "time trig":dbl, "time trig 2":dbl, "DC":dbl, "trigger detected?":bool, "FFT amplitude mean":dbl}
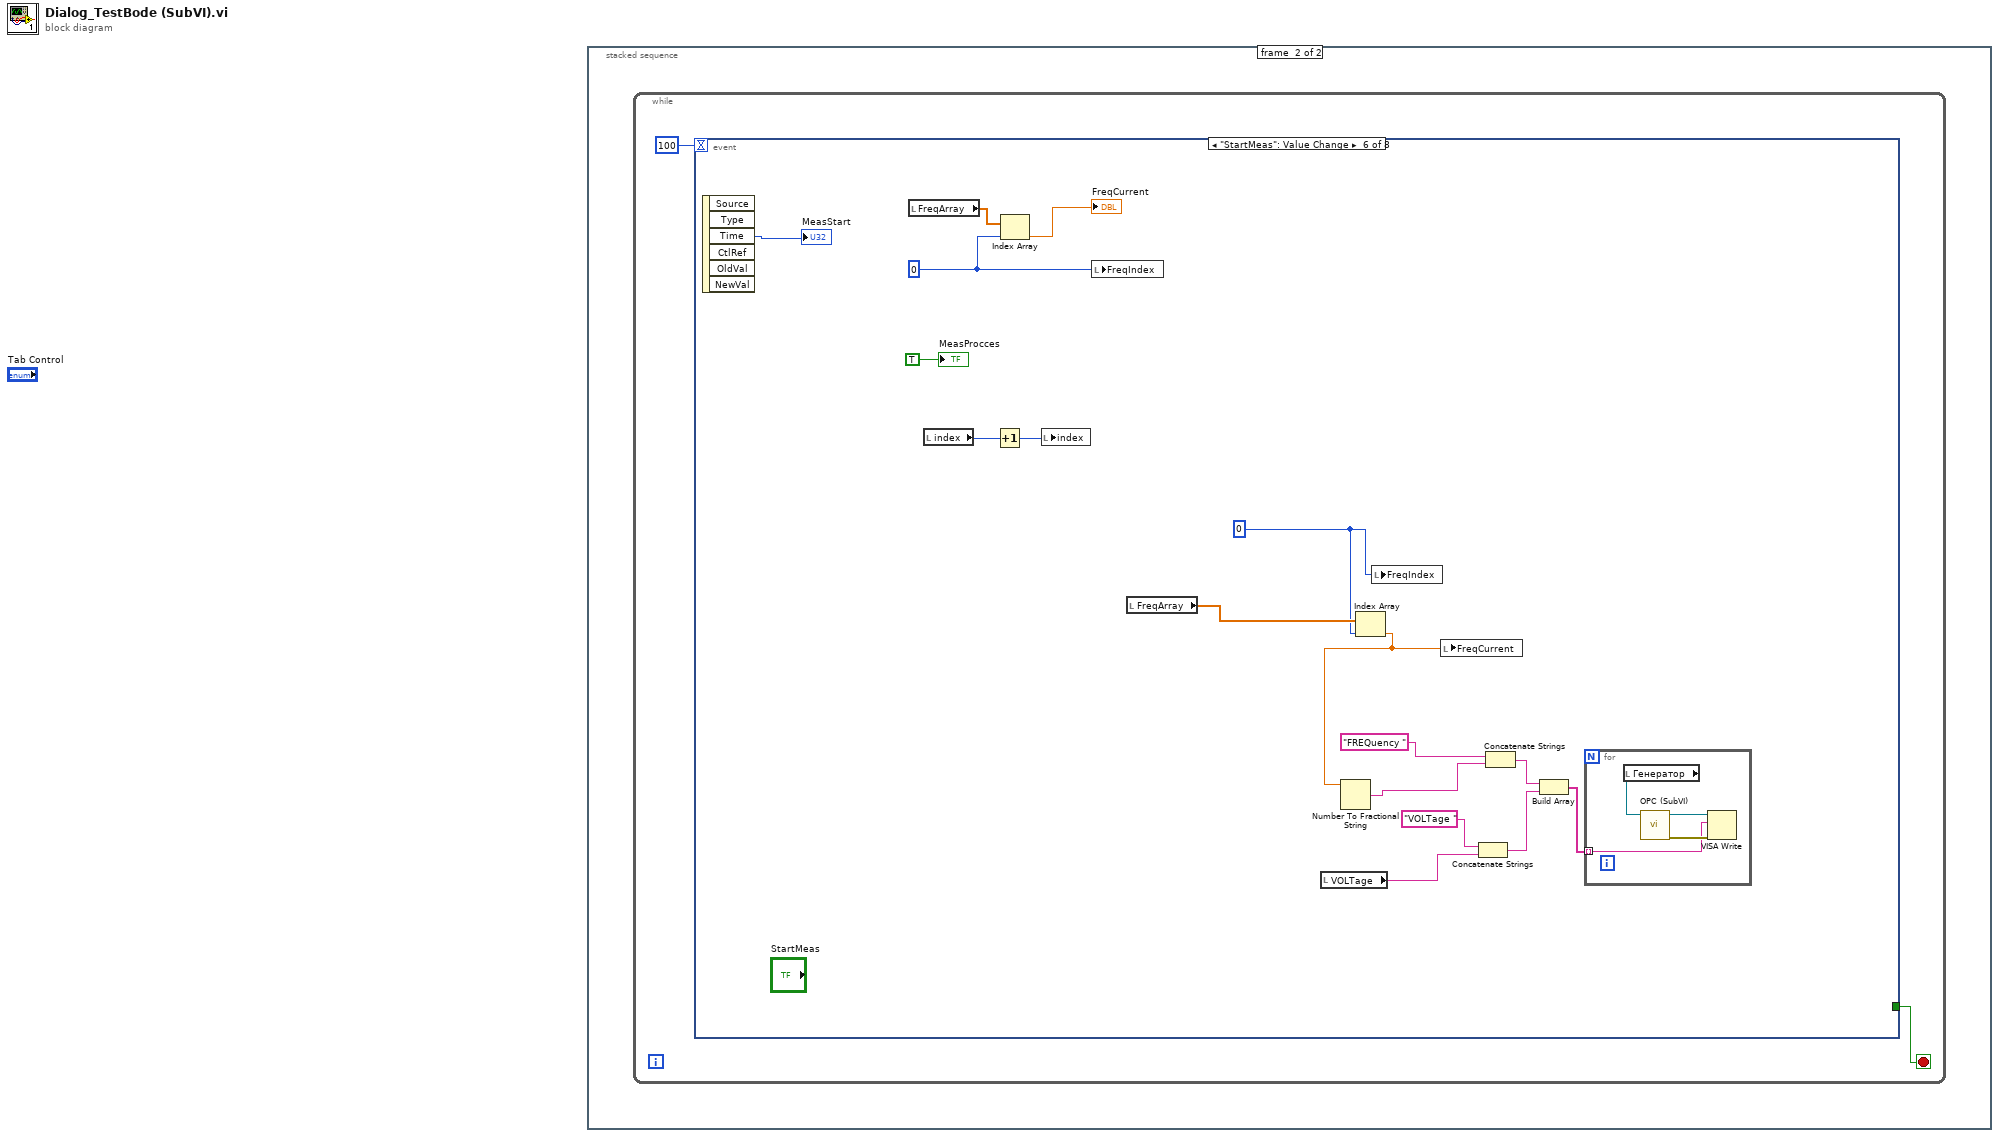
[diagram p0: block diagram]
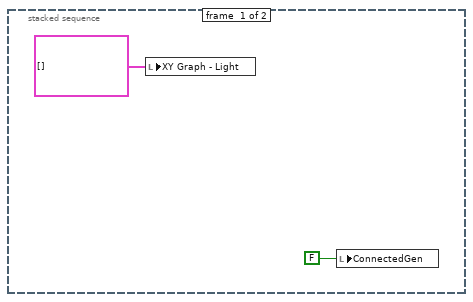
[diagram p2: hidden frame]
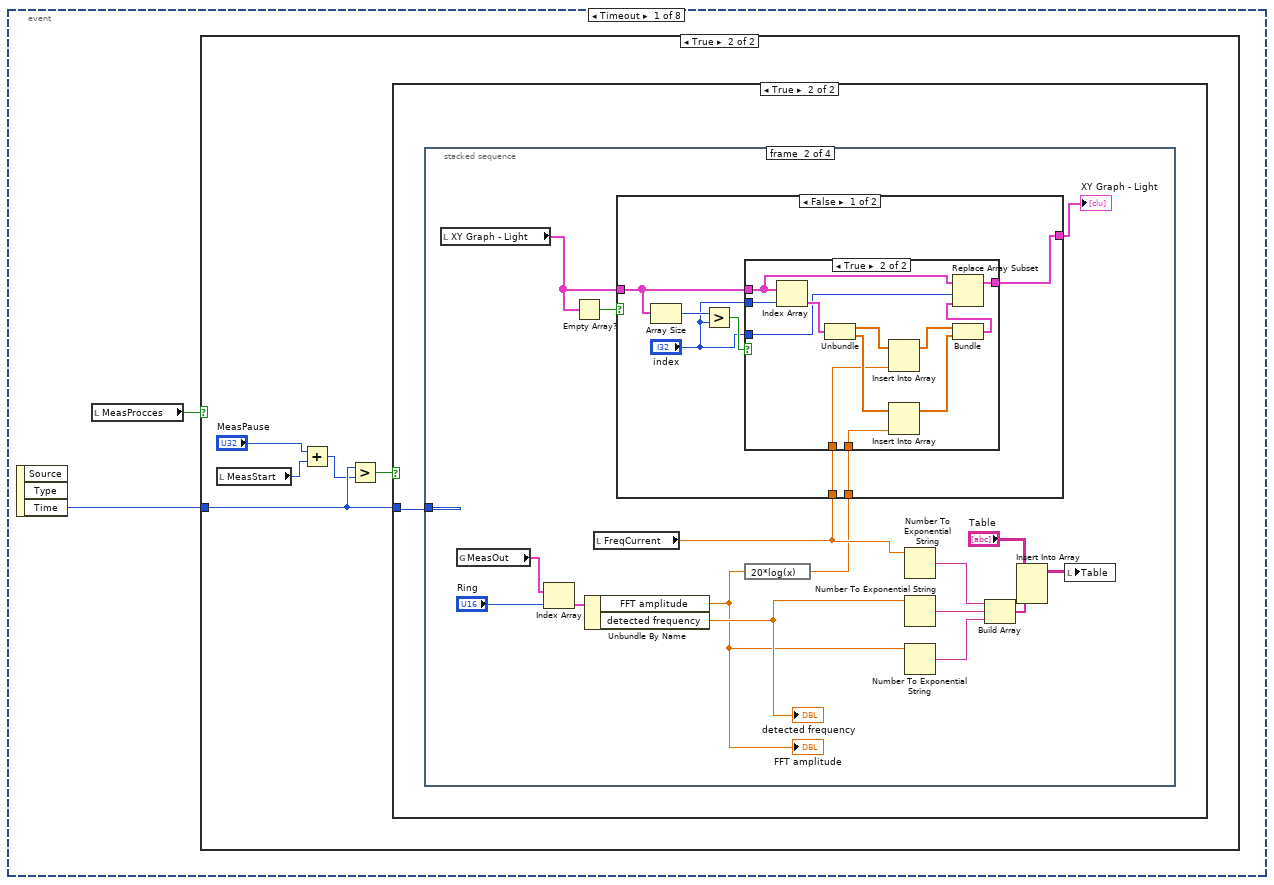
[diagram p3: hidden frame]
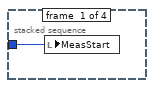
[diagram p6: hidden frame]
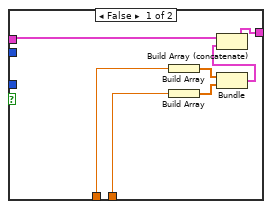
[diagram p7: hidden frame]
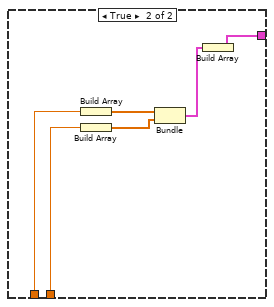
[diagram p8: hidden frame]
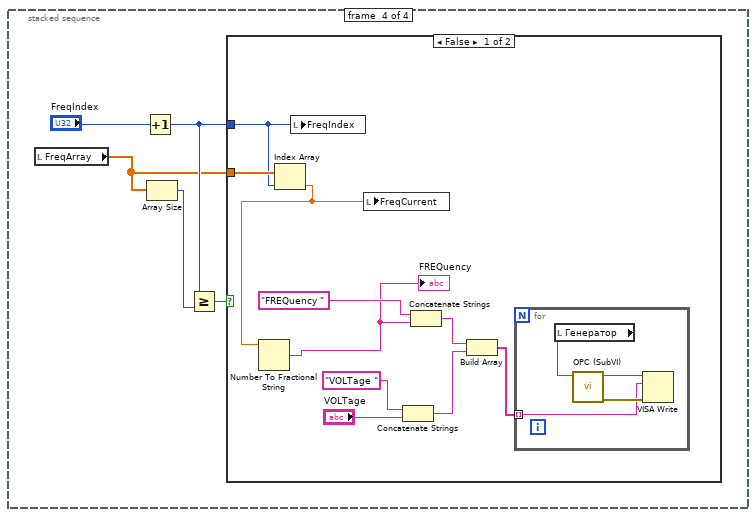
[diagram p10: hidden frame]
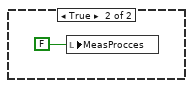
[diagram p11: hidden frame]
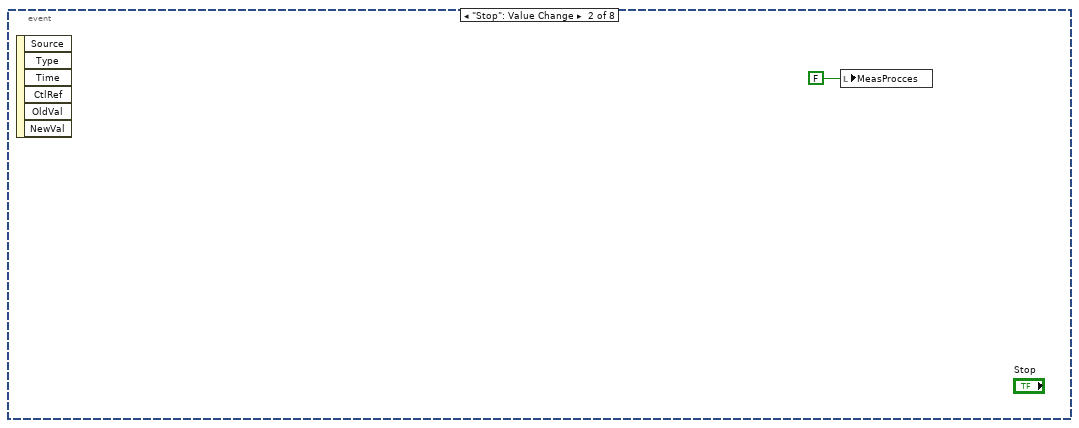
[diagram p12: hidden frame]
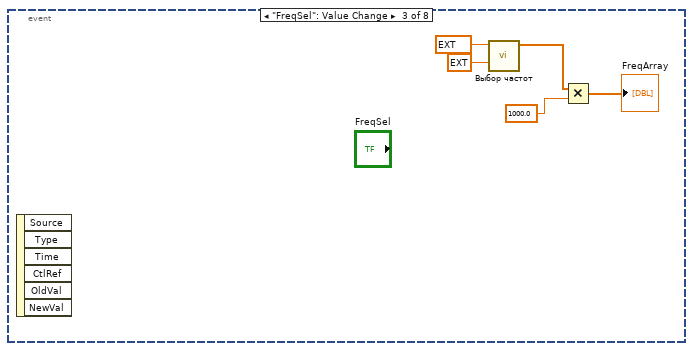
[diagram p13: hidden frame]
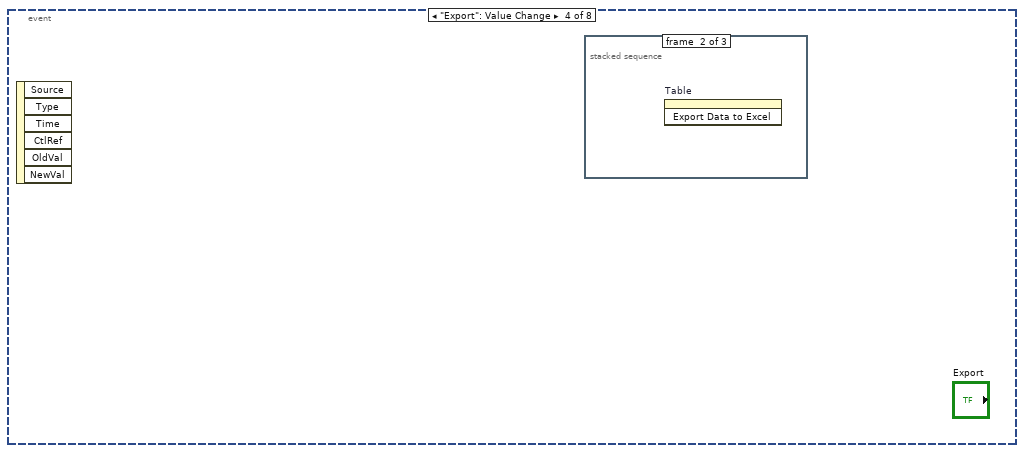
[diagram p14: hidden frame]
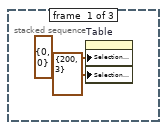
[diagram p15: hidden frame]
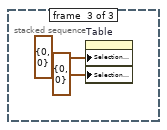
[diagram p16: hidden frame]
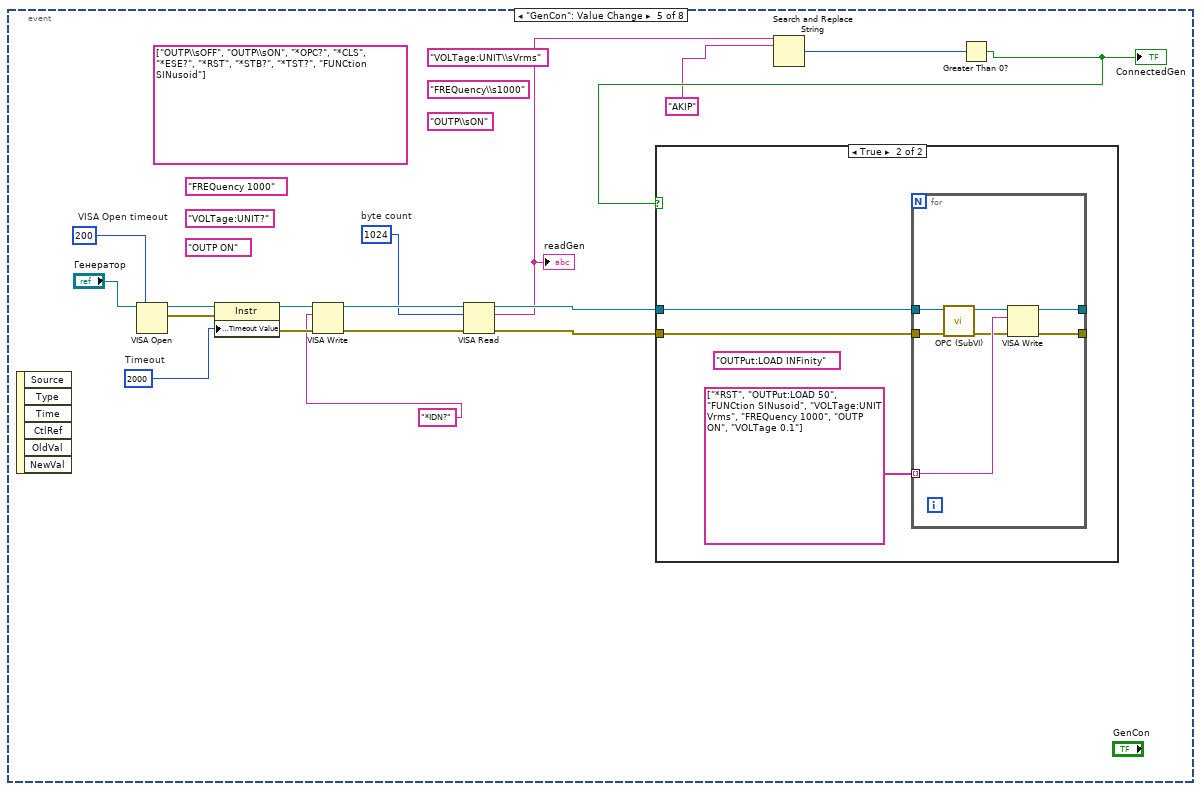
[diagram p17: hidden frame]
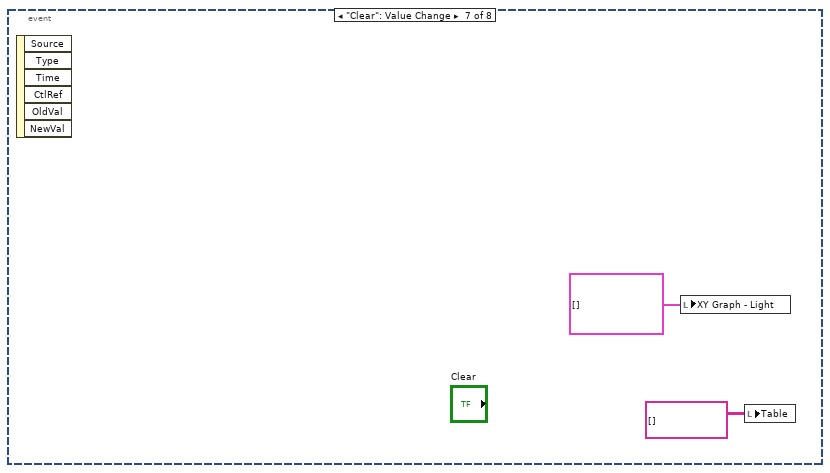
[diagram p19: hidden frame]
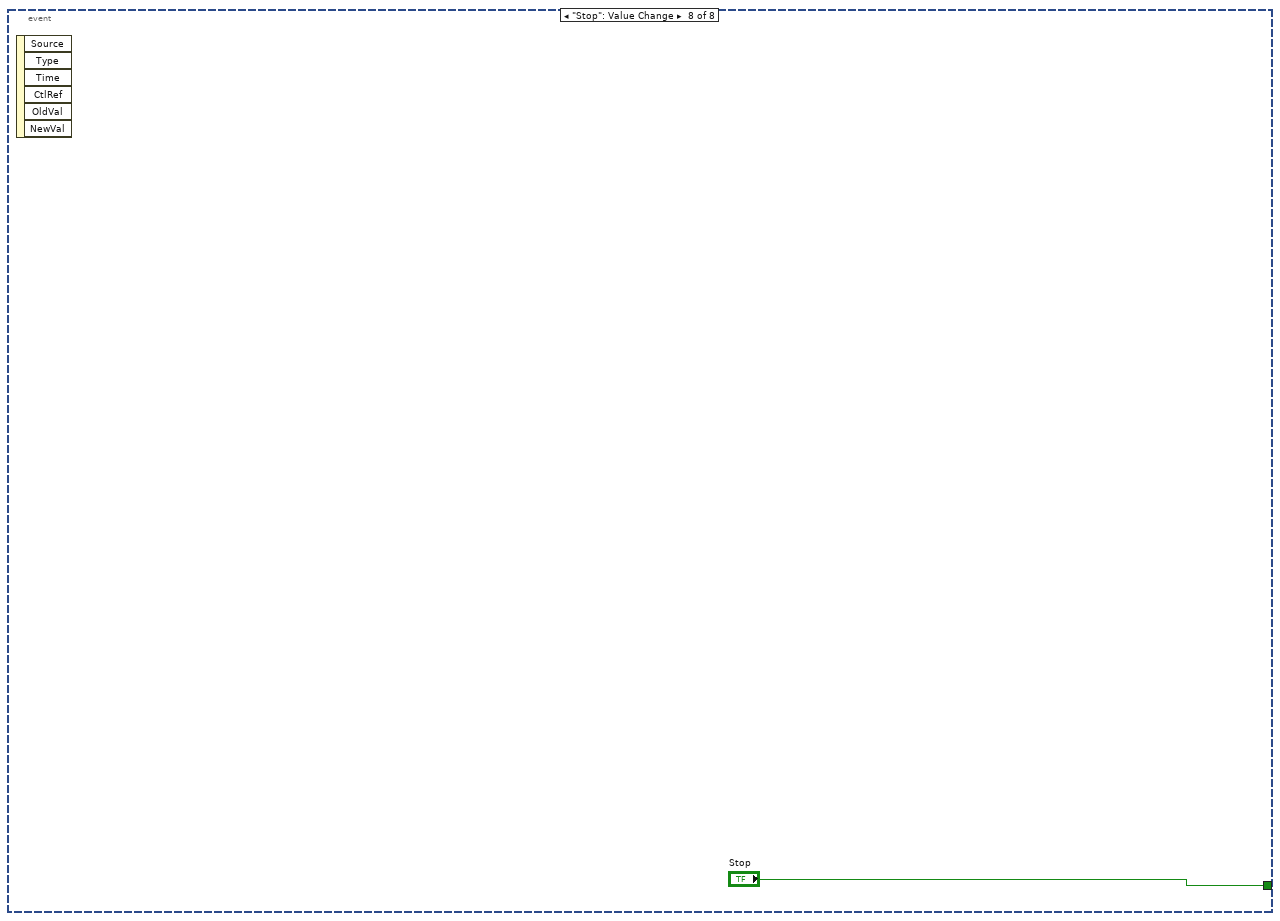
[diagram p20: hidden frame]
diagram:
  n1 = stacked-sequence {
    frame #0 {
      n2 = local write "XY Graph - Light"(cluster{dbl[], dbl[]}[] [] ("XY Graph - Light")) -> ()
      n3 = local write "ConnectedGen"(FALSE ("ConnectedGen")) -> ()
    }
    frame #1 {
      n4 = while {
        stop <- w3 stop-if-true
        n5 = event shown="[5] \"StartMeas\": Value Change" {
          selector: _ -> [_ _ _ _ _ _ _ _]
          dyn-events: _ -> [_ _ _ _ _ _ _ _]
          timeout: 100 -> [_ _ _ _ _ _ _ _]
          tunnel: [_ _ _ _ _ _ _ "Stop"] -> w3
          event Timeout {
            n6 = event-data() -> ("Time"=w5:u32)  [unwired: 1 in, 2 out]
            n7 = local read "MeasProcces"() -> (w6:bool)
            n8 = case shown="True" w6 {
              tunnel: w5 -> [_ w8]
              frame False {
              }
              frame True {
                n9 = local read "MeasStart"() -> (w10:u32)
                n10 = Add(x="MeasPause", y=w10) -> (x+y=w7:u32)
                n11 = Greater?(x=w8, y=w7) -> (0:w9:bool)
                n12 = case shown="True" w9 {
                  tunnel: w8 -> [_ w12]
                  frame False {
                  }
                  frame True {
                    n13 = stacked-sequence {
                      tunnel: w12 -> [w13 _ _ _]
                      frame #0 {
                        n14 = local write "MeasStart"(w13) -> ()
                      }
                      frame #1 {
                        n15 = local read "XY Graph - Light"() -> (w14:cluster{dbl[], dbl[]}[])
                        n16 = global read "Global_SNK3_HF.vi" "MeasOut"() -> (w28:T2[])
                        n17 = Index Array(array=w28, index="Ring") -> (element=w29:T2)
                        n18 = Empty Array?(array=w14) -> (empty?=w15:bool)
                        n19 = Unbundle By Name(w29) -> ("FFT amplitude"=w17:dbl, "detected frequency"=w18:dbl)
                        "FFT amplitude" <- w17
                        "detected frequency" <- w18
                        n20 = local read "FreqCurrent"() -> (w19:dbl)
                        n21 = expression code="20*log(x)"(w17) -> (w16:dbl)
                        n22 = case shown="False" w15 {
                          tunnel: [w30 w56] -> w20
                          tunnel: w19 -> [w36 w61]
                          tunnel: w16 -> [w35 w60]
                          tunnel: w14 -> [w34 _]
                          frame False {
                            n23 = Array Size(array=w34) -> (size(s)=w33:i32)
                            n24 = Greater?(x=w33, y="index") -> (0:w32:bool)
                            n25 = case shown="True" w32 {
                              tunnel: w36 -> [w43 w50]
                              tunnel: w35 -> [w42 w49]
                              tunnel: w34 -> [w39 w44]
                              tunnel: "index" -> [_ w48]
                              tunnel: "index" -> [_ w47]
                              tunnel: [w37 w45] -> w30
                              frame False {
                                n26 = Build Array(w43) -> (w41:dbl[])
                                n27 = Build Array(w42) -> (w40:dbl[])
                                n28 = Bundle(w41, w40) -> (w38:cluster{dbl[], dbl[]})  [unwired: 1 in]
                                n29 = Build Array (concatenate)(w39, w38) -> (w37:cluster{dbl[], dbl[]}[])
                              }
                              frame True {
                                n30 = Index Array(array=w44, index=w48) -> (element=w51:cluster{dbl[], dbl[]})
                                n31 = Unbundle(w51) -> (w52:dbl[], w55:dbl[])
                                n32 = Insert Into Array(array=w52, new element=w50) -> (w53:dbl[])  [unwired: 1 in]
                                n33 = Insert Into Array(array=w55, new element=w49) -> (w54:dbl[])  [unwired: 1 in]
                                n34 = Bundle(w53, w54) -> (w46:cluster{dbl[], dbl[]})  [unwired: 1 in]
                                n35 = Replace Array Subset(array=w44, new element=w46, index=w47) -> (w45:cluster{dbl[], dbl[]}[])
                              }
                            }
                          }
                          frame True {
                            n36 = Build Array(w61) -> (w59:dbl[])
                            n37 = Build Array(w60) -> (w58:dbl[])
                            n38 = Bundle(w59, w58) -> (w57:cluster{dbl[], dbl[]})  [unwired: 1 in]
                            n39 = Build Array(w57) -> (w56:cluster{dbl[], dbl[]}[])
                          }
                        }
                        "XY Graph - Light" <- w20
                        n40 = Number To Exponential String(number=w19) -> (E-format string=w26:string)  [unwired: 3 in]
                        n41 = Number To Exponential String(number=w18) -> (E-format string=w25:string)  [unwired: 3 in]
                        n42 = Number To Exponential String(number=w17) -> (E-format string=w24:string)  [unwired: 3 in]
                        n43 = Build Array(w26, w25, w24) -> (w22:string[])
                        n44 = Insert Into Array(array="Table", new element=w22) -> (w21:string[][])  [unwired: 2 in]
                        n45 = local write "Table"(w21) -> ()
                      }
                      frame #2 {
                      }
                      frame #3 {
                        n46 = local read "FreqArray"() -> (w62:dbl[])
                        n47 = Increment(x="FreqIndex") -> (x+1=w64:u32)
                        n48 = Array Size(array=w62) -> (size(s)=w63:i32)
                        n49 = Greater Or Equal?(x=w64, y=w63) -> (x >= y?=w66:bool)
                        n50 = case shown="False" w66 {
                          tunnel: w64 -> [w68 _]
                          tunnel: w62 -> [w69 _]
                          frame False {
                            n51 = Index Array(array=w69, index=w68) -> (element=w67:dbl)
                            n52 = Number To Fractional String(number=w67) -> (F-format string=w70:string)  [unwired: 3 in]
                            "FREQuency" <- w70
                            n53 = local write "FreqIndex"(w68) -> ()
                            n54 = local write "FreqCurrent"(w67) -> ()
                            n55 = Concatenate Strings("VOLTage " ("string"), "VOLTage") -> (w75:string)
                            n56 = Concatenate Strings("FREQuency " ("string"), w70) -> (w73:string)
                            n57 = Build Array(w73, w75) -> (w74:string[])
                            n58 = for {
                              tunnel: w74 -> [w77] mode=indexing
                              n59 = local read "Генератор"() -> (w78:refnum<visa-resource-name>)
                              n60 = call "OPC (SubVI).vi"("VISA Refnum in"=w78) -> ("error out"=w80:errorcluster, "VISA Refnum out"=w79:refnum<visa-resource-name>)  [unwired: 9 in]
                              n61 = VISA Write(VISA resource name=w79, write buffer=w77, error in (no error)=w80) -> ()  [unwired: 3 out]
                            }
                          }
                          frame True {
                            n62 = local write "MeasProcces"(FALSE ("MeasProcces")) -> ()
                          }
                        }
                      }
                    }
                  }
                }
              }
            }
          }
          event "Stop": Value Change {
            n63 = event-data() -> ()  [unwired: 1 in, 6 out]
            n64 = local write "MeasProcces"(FALSE ("MeasProcces")) -> ()
          }
          event "FreqSel": Value Change {
            n65 = event-data() -> ()  [unwired: 1 in, 6 out]
            n66 = call "Выбор частот.vi"("Нижняя частота"=ext 100.0, "Верхняя частота"=ext 20000.0) -> ("Array"=w85:dbl[])  [unwired: 9 in]
            n67 = Multiply(x=w85, y=1000.0) -> (x*y=→"FreqArray":dbl[])
          }
          event "Export": Value Change {
            n68 = event-data() -> ()  [unwired: 1 in, 6 out]
            n69 = stacked-sequence {
              frame #0 {
                n70 = property on="Table" class="Tbl (strict)"("Selection Start"=T1 {"Row"=0, "Column"=0}, "Selection Size"=T1 {"Row"=200, "Column"=3}) -> ()  [unwired: 2 in, 2 out]
              }
              frame #1 {
                n71 = invoke on="Table" class="Tbl (strict)" method="Export Data to Excel"() -> ()  [unwired: 3 in, 3 out]
              }
              frame #2 {
                n72 = property on="Table" class="Tbl (strict)"("Selection Start"=T1 {"Row"=0, "Column"=0}, "Selection Size"=T1 {"Row"=0, "Column"=0}) -> ()  [unwired: 2 in, 2 out]
              }
            }
          }
          event "GenCon": Value Change {
            (unwired) "OUTP ON" ("string")
            (unwired) "FREQuency 1000" ("string")
            (unwired) "VOLTage:UNIT?" ("string")
            (unwired) "OUTP\\sON" ("string")
            (unwired) "VOLTage:UNIT\\sVrms" ("string")
            (unwired) "FREQuency\\s1000" ("string")
            (unwired) string[] ["OUTP\\sOFF", "OUTP\\sON", "*OPC?", "*CLS", "*ESE?", "*RST", "*STB?", "*TST?", "FUNCtion SINusoid"]
            w92 = u32 1024  # byte count
            w94 = u32 2000  # Timeout
            w93 = u32 200  # VISA Open timeout
            n73 = event-data() -> ()  [unwired: 1 in, 6 out]
            n74 = VISA Open(timeout (0)=w93, VISA resource name="Генератор") -> (VISA resource name=w108:refnum<visa-resource-name>, error out=w107:errorcluster)  [unwired: 3 in]
            n75 = property class="Instr"(reference=w108, error in=w107, "General Settings:Timeout Value"=w94) -> (reference out=w106:refnum<visa-resource-name>, error out=w105:errorcluster)
            n76 = VISA Write(VISA resource name=w106, write buffer="*IDN?" ("string"), error in (no error)=w105) -> (VISA resource name out=w104:refnum<visa-resource-name>, error out=w103:errorcluster)  [unwired: 1 out]
            n77 = VISA Read(VISA resource name=w104, byte count=w92, error in (no error)=w103) -> (VISA resource name out=w101:refnum<visa-resource-name>, read buffer=w98:string, error out=w100:errorcluster)  [unwired: 1 out]
            "readGen" <- w98
            n78 = Search and Replace String(input string=w98, search string="AKIP") -> (number of replacements=w99:i32)  [unwired: 6 in, 3 out]
            n79 = Greater Than 0?(x=w99) -> (x > 0?=w97:bool)
            "ConnectedGen" <- w97
            n80 = case shown="True" w97 {
              tunnel: w101 -> [_ w111]
              tunnel: w100 -> [_ w110]
              frame False {
              }
              frame True {
                (unwired) "OUTPut:LOAD INFinity" ("string")
                n81 = for {
                  tunnel: w111 -> [w115]
                  tunnel: w110 -> [w114]
                  tunnel: string[] ["*RST", "OUTPut:LOAD 50", "FUNCtion SINusoid", "VOLTage:UNIT Vrms", "FREQuency 1000", "OUTP ON", "VOLTage 0.1"] -> [w118] mode=indexing
                  tunnel: [w117] -> _
                  tunnel: [w116] -> _
                  n82 = call "OPC (SubVI).vi"("error in (no error)"=w114, "VISA Refnum in"=w115) -> ("error out"=w113:errorcluster, "VISA Refnum out"=w112:refnum<visa-resource-name>)  [unwired: 8 in]
                  n83 = VISA Write(VISA resource name=w112, write buffer=w118, error in (no error)=w113) -> (VISA resource name out=w117:refnum<visa-resource-name>, error out=w116:errorcluster)  [unwired: 1 out]
                }
              }
            }
          }
          event "StartMeas": Value Change {
            w122 = 0
            w131 = u32 0 ("FreqIndex")
            n84 = event-data() -> ("Time"=→"MeasStart":u32)  [unwired: 1 in, 5 out]
            n85 = local read "FreqArray"() -> (w133:dbl[])
            n86 = local read "index"() -> (w130:i32)
            n87 = Increment(x=w130) -> (x+1=w129:i32)
            n88 = Index Array(array=w133, index=w131) -> (element=→"FreqCurrent":dbl)
            n89 = local write "index"(w129) -> ()
            n90 = local write "FreqIndex"(w131) -> ()
            n91 = local read "FreqArray"() -> (w123:dbl[])
            n92 = local read "VOLTage"() -> (w119:string)
            n93 = Index Array(array=w123, index=w122) -> (element=w128:dbl)
            n94 = Number To Fractional String(number=w128) -> (F-format string=w127:string)  [unwired: 3 in]
            n95 = local write "FreqIndex"(w122) -> ()
            n96 = local write "FreqCurrent"(w128) -> ()
            n97 = Concatenate Strings("VOLTage " ("string"), w119) -> (w124:string)
            n98 = Concatenate Strings("FREQuency " ("string"), w127) -> (w126:string)
            n99 = Build Array(w126, w124) -> (w125:string[])
            n100 = for {
              tunnel: w125 -> [w136] mode=indexing
              n101 = local read "Генератор"() -> (w137:refnum<visa-resource-name>)
              n102 = call "OPC (SubVI).vi"("VISA Refnum in"=w137) -> ("error out"=w139:errorcluster, "VISA Refnum out"=w138:refnum<visa-resource-name>)  [unwired: 9 in]
              n103 = VISA Write(VISA resource name=w138, write buffer=w136, error in (no error)=w139) -> ()  [unwired: 3 out]
            }
            "MeasProcces" <- TRUE ("MeasProcces")
          }
          event "Clear": Value Change {
            n104 = event-data() -> ()  [unwired: 1 in, 6 out]
            n105 = local write "XY Graph - Light"(cluster{dbl[], dbl[]}[] [] ("XY Graph - Light")) -> ()
            n106 = local write "Table"(string[][] [] ("Table")) -> ()
          }
          event "Stop": Value Change {
            n107 = event-data() -> ()  [unwired: 1 in, 6 out]
          }
        }
      }
    }
  }
